vi "action.vi"(0 "HGF_Device_Reset":refnum<class "HGF_Device_Reset.lvclass">, 2 "HGF_Visitable":refnum<class "HGF_Visitable.lvclass">, 5 "error in (no error)":errorcluster) -> (14 "dup HGF_Device_Reset":refnum<class "HGF_Device_Reset.lvclass">, 16 "dup HGF_Visitable":refnum<class "HGF_Visitable.lvclass">, 19 "error out":errorcluster)   [LabVIEW 2014, in "HGF_DeviceBaseClasses.lvlib" / "HGF_Device_Reset.lvclass"]
doc: "This is a dynamic dispatch VI that is called from Visitor.visit(). It will call member VIs of Visitable to perform the requested action which means: calling public methods of Visitable child class.\n\n<B>Hint:</B> This method is abstract and need to be implemented by child classes."
uses:
  HGF_Device_Reset.lvclass
  HGF_DeviceBase/HGF_DeviceBase.lvclass
  HGF_BaseClasses/HGF_Visitable/HGF_Visitable.lvclass
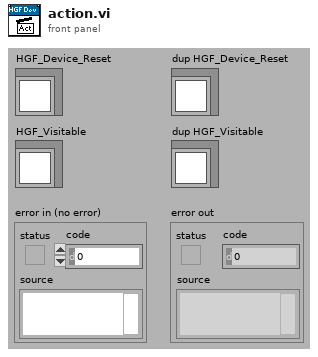
[diagram p1: front panel]
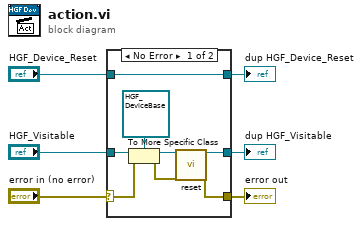
[diagram p0: block diagram]
diagram:
  n1 = case shown="No Error" "error in (no error)" {
    selector: "error in (no error)" -> [w10 w16]
    tunnel: "HGF_Visitable" -> [w14 w17]
    tunnel: [w11 w17] -> w5
    tunnel: [w8 w16] -> w3
    tunnel: [w7 w15] -> w2
    tunnel: "HGF_Device_Reset" -> [w7 w15]
    frame No Error {
      n2 = To More Specific Class(target class=refnum<class "HGF_DeviceBase.lvclass"> refnum ("HGF_DeviceBaseClasses.lvlib:HGF_DeviceBase.lvclass"), reference=w14, error in=w10) -> (specific class reference=w12:refnum<class "HGF_DeviceBase.lvclass">, error out=w9:errorcluster)
      n3 = call-dynamic "reset.vi"("HGF_DeviceBase"=w12, "error in (no error)"=w9) -> ("dup HGF_DeviceBase"=w11:refnum<class "HGF_DeviceBase.lvclass">, "error out"=w8:errorcluster)  [unwired: 16 out]
    }
    frame Error {
    }
  }
  "error out" <- w3
  "dup HGF_Device_Reset" <- w2
  "dup HGF_Visitable" <- w5
